vi "Update_c_ForAmplitudeFeedback.vi"(7 "Reset":bool=TRUE, 8 "input valid":bool=TRUE, 10 "delta_c":fxp<+/-,32,21>) -> (0 "output valid":bool, 3 "c out":fxp<+/-,32,21>)   [LabVIEW 2013]
doc: "Increases Fi with Fi_delta. Also wraps Fi to the range [0, 2*Pi]"
uses:
  <vilib>/rvi/FXPMathLib/FxpAdd/XNode/nifxpmath_Add.xnode
  <vilib>/rvi/FXPMathLib/sim/FxpSim.dll
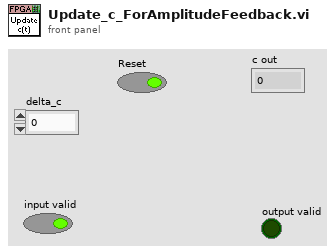
[diagram p1: front panel]
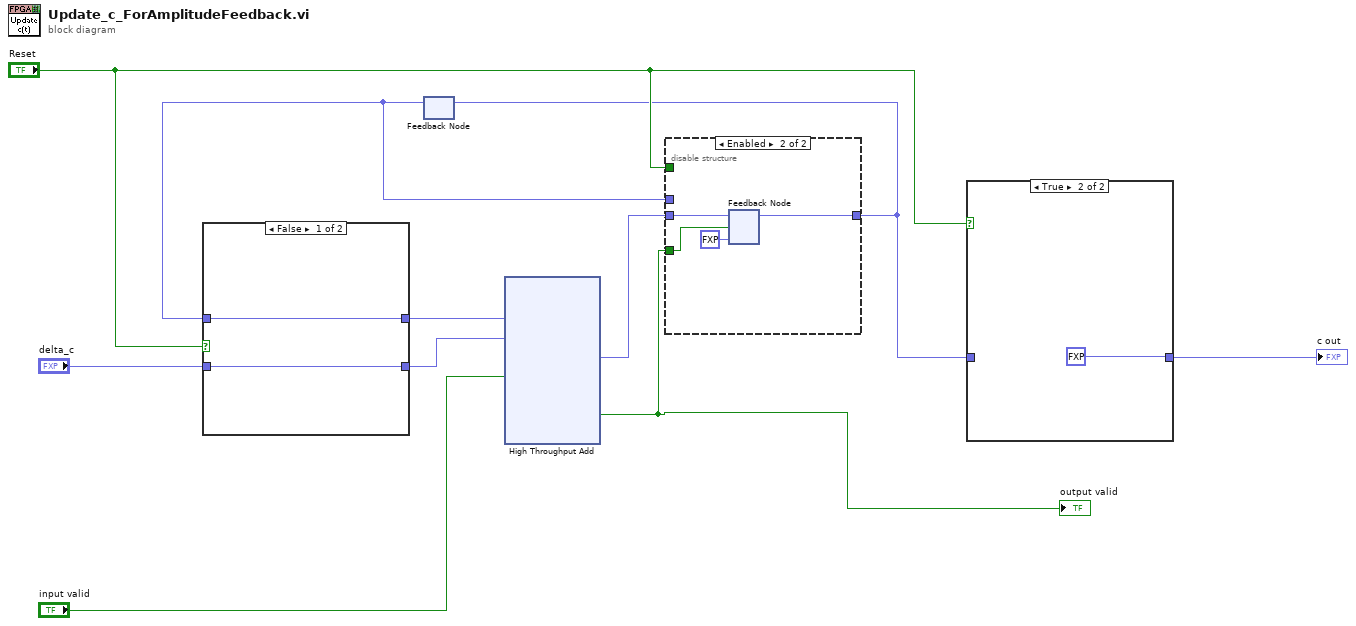
[diagram p0: block diagram]
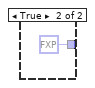
[diagram p4: hidden frame]
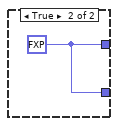
[diagram p6: hidden frame]
diagram:
  n1 = feedback #1() -> (w3:fxp<+/-,32,21>)  [unwired: 1 in]
  n2 = case shown="False" "Reset" {
    tunnel: [w11 w13] -> w10
    tunnel: "delta_c" -> [w12 _]
    tunnel: [w12 w13] -> w7
    tunnel: w3 -> [w11 _]
    frame False {
    }
    frame True {
      w13 = fxp<+/-,32,21> 0.0 ("x+y")
    }
  }
  n3 = xnode "High Throughput Add"("x"=w10, "y"=w7, "input valid"="input valid") -> ("x+y"=w4:fxp<+/-,32,21>, "output valid"=w5:bool)  [unwired: 1 in, 1 out]
  "output valid" <- w5
  n4 = disable-structure shown="Enabled" {
    disable-tunnel: w5 -> [w18 w29]
    disable-tunnel: w4 -> [w17 w28]
    disable-tunnel: w3 -> [w16 _]
    disable-tunnel: "Reset" -> [w15 _]
    disable-tunnel: [w14 w27] -> w1
    frame Disabled {
      n5 = case shown="False" w15 {
        tunnel: w18 -> [w22 _]
        tunnel: w17 -> [w21 _]
        tunnel: [w20 fxp<+/-,32,21> 0.0 ("x+y")] -> w14
        tunnel: w16 -> [w19 _]
        frame False {
          n6 = case shown="False" w22 {
            tunnel: w21 -> [_ w24]
            tunnel: [w23 w24] -> w20
            tunnel: w19 -> [w23 _]
            frame False {
            }
            frame True {
            }
          }
        }
        frame True {
        }
      }
    }
    frame Enabled {
      n7 = feedback #2(fxp<+/-,32,21> 0.0 ("x+y")) -> (w27:fxp<+/-,32,21>)
      n8 = feedback-in #2(w28, w29) -> ()
    }
  }
  n9 = feedback-in #1(w1) -> ()
  n10 = case shown="True" "Reset" {
    tunnel: [w30 fxp<+/-,32,21> 0.0 ("c out")] -> w6
    tunnel: w1 -> [w30 _]
    frame False {
    }
    frame True {
    }
  }
  "c out" <- w6
